vi "Config.vi"(0 "Resources in":T2 {"ZI ModHandle"."ModHandle" format="0x%08x"; "ZI ModHandle"."Conn" format="0x%08x"; "ZI Handle"."Handle" format="0x%08x"; "ZI Handle"."Conn" format="0x%08x"}, 1 "Config files paths":T5={"ZI config file (.ini)"="Config_Ver_2\\Zurich_params.ini", "Keithley config file (.ini)"="Config_Ver_2\\Keithley_params.ini", "DAQ config file (.ini)"="Config_Ver_2\\pulse_sequence_DAQ.ini"}, 11 "error in":errorcluster) -> (4 "Resources out":T2 {"ZI ModHandle"."ModHandle" format="0x%08x"; "ZI ModHandle"."Conn" format="0x%08x"; "ZI Handle"."Handle" format="0x%08x"; "ZI Handle"."Conn" format="0x%08x"}, 6 "Final Sending Data":u32[](array[numeric]), 8 "Time Unit":T1(ring), 12 "Period (s)":dbl=5.0, 13 "Sample Numbers":u32=20000000, 14 "Sample Frequency (Hz)":u32=1000000, 15 "error out":errorcluster)   [LabVIEW 2021]
uses:
  Main/Ver_2/Config_File_Paths_v2.ctl
  Main/Ver_2/Resources_v2.ctl
  <instrlib>/Zurich Instruments LabOne/Public/ziTypeHandle.ctl
  <instrlib>/Zurich Instruments LabOne/Public/Modules/ziTypeModHandle.ctl
  <instrlib>/Zurich Instruments LabOne/Zurich Instruments LabOne.lvlib
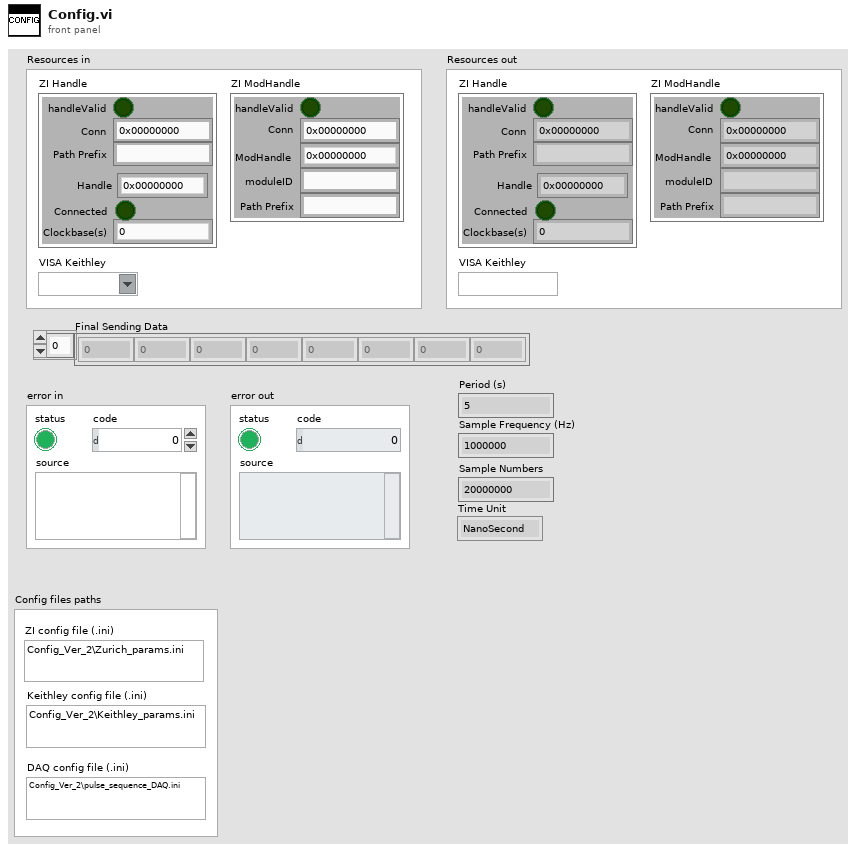
[diagram p1: front panel]
types:
  T1 = enum16{"NanoSecond", "MicroSecond", "MilliSecond"}
  T2 = typedef "Resources_v2.ctl" = cluster{"ZI Handle":T3, "ZI ModHandle":T4, "VISA Keithley":refnum<visa-resource-name>}
  T3 = typedef "Zurich Instruments LabOne.lvlib/ziTypeHandle.ctl" = cluster{"handleValid":bool, "Conn":u64, "Path Prefix":string, "Handle":u64, "Clockbase(s)":dbl, "Connected":bool}
  T4 = typedef "Zurich Instruments LabOne.lvlib/ziTypeModHandle.ctl" = cluster{"handleValid":bool, "Conn":u64, "ModHandle":u64, "moduleID":string, "Path Prefix":string}
  T5 = typedef "Config_File_Paths_v2.ctl" = cluster{"ZI config file (.ini)":string, "Keithley config file (.ini)":string, "DAQ config file (.ini)":string}
  T6 = typedef "DAQ_Control_1.ctl" = cluster{"Port 2/line 6":cluster{"Timing 22":dbl[]}, "Port 2/line 5":cluster{"Timing 21":dbl[]}, "Port 2/line 4":cluster{"Timing 20":dbl[]}, "Port 2/line 3":cluster{"Timing 19":dbl[]}, "Port 2/line 2":cluster{"Timing 18":dbl[]}, "Port 2/line 1":cluster{"Timing 17":dbl[]}, "Port 2/line 0":cluster{"Timing 16":dbl[]}, "Port 1/line 7":cluster{"Timing 15":dbl[]}, "Port 1/line 6":cluster{"Timing 14":dbl[]}, "Port 1/line 5":cluster{"Timing 13":dbl[]}, "Port 1/line 4":cluster{"Timing 12":dbl[]}, "Port 1/line 3":cluster{"Timing 11":dbl[]}, "Port 1/line 2":cluster{"Timing 10":dbl[]}, "Port 1/line 1":cluster{"Timing 9":dbl[]}, "Port 1/line 0":cluster{"Timing 8":dbl[]}, "Port 0/line 7":cluster{"Timing 7\n":dbl[]}, "Port 0/line 6":cluster{"Timing 6\n":dbl[]}, "Port 0/line 5":cluster{"Timing 5\n":dbl[]}, "Port 0/line 4":cluster{"Timing 4\n":dbl[]}, "Port 0/line 3":cluster{"Timing 3\n":dbl[]}, "Port 0/line 2":cluster{"Timing 2":dbl[]}, "Port 0/line 1":cluster{"Timing 1\n":dbl[]}, "Port 0/line 0":cluster{"Timing 0":dbl[]}}
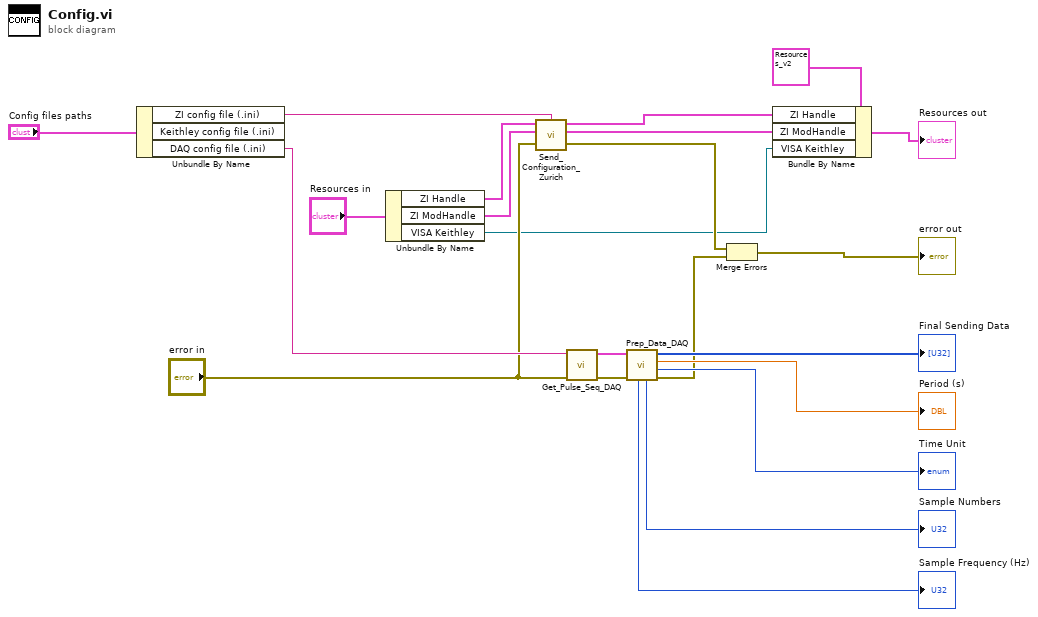
[diagram p0: block diagram]
diagram:
  n1 = Unbundle By Name("Config files paths") -> ("ZI config file (.ini)"=w16:string, "DAQ config file (.ini)"=w11:string)  [unwired: 1 out]
  n2 = Unbundle By Name("Resources in") -> ("ZI Handle"=w22:T3, "ZI ModHandle"=w21:T4, "VISA Keithley"=w1:refnum<visa-resource-name>)
  n3 = call "Send_Configuration_Zurich.vi"("Filename (.ini)"=w16, "Handle In"=w22, "ModHandle In"=w21, "error in"="error in") -> ("Handle Out"=w19:T3, "ModHandle Out"=w20:T4, "error out"=w18:errorcluster)  [unwired: 1 in]
  n4 = call "Get_Pulse_Seq_DAQ.vi"("error in"="error in", "Filename (ini)"=w11) -> ("error out"=w9:errorcluster, "data"=w10:T6)  [unwired: 8 in]
  n5 = call "Prep_Data_DAQ.vi"("Error  in"=w9, "Sequence"=w10) -> ("Error out"=w2:errorcluster, "Time Unit"=→"Time Unit":T1, "Period (s )=Sample Numbers / Sample Frequency"=→"Period (s)":dbl, "Final Sending Data"=→"Final Sending Data":u32[], "Sample Numbers"=→"Sample Numbers":u32, "Sample Frequency (Hz)"=→"Sample Frequency (Hz)":u32)  [unwired: 4 in]
  n6 = Merge Errors(w18, w2) -> (→"error out":errorcluster)
  n7 = Bundle By Name(cluster=T2 {"ZI Handle"={"handleValid"=FALSE, "Conn"=0, "Path Prefix"="", "Handle"=0, "Clockbase(s)"=0.0, "Connected"=FALSE}, "ZI ModHandle"={"handleValid"=FALSE, "Conn"=0, "ModHandle"=0, "moduleID"="", "Path Prefix"=""}, "VISA Keithley"=""} ("Resources"), "ZI Handle"=w19, "ZI ModHandle"=w20, "VISA Keithley"=w1) -> (→"Resources out":T2)
